vi "Accel Sensitivity.vi"(8 "error in (no error)":errorcluster, 11 "Accel Sensitivities":dbl[](array[numeric])) -> (0 "error out":errorcluster)   [LabVIEW 2018, in "PC UDP Writer.lvlib"]
doc: "This subVI enqueues the named action in to the communications queue along with the input data."
uses:
  PC UDP Writer.lvlib
  Private Controls/Module Data.ctl
  Private Controls/Module Action.ctl
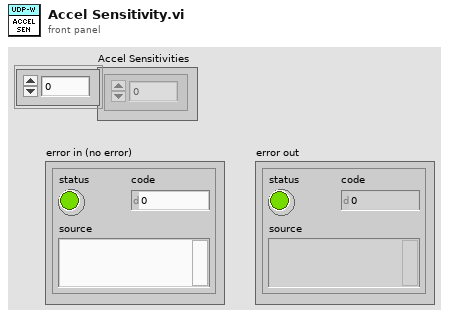
[diagram p1: front panel]
types:
  T1 = typedef "PC UDP Writer.lvlib/Module Data.ctl" = cluster{"Data":variant, "Action":T2}
  T2 = typedef "PC UDP Writer.lvlib/Module Action.ctl" = enum8{"Init", "Waterfall Select", "Bleed Fuel", "Fuel Pressure Reg", "ECS Demand", "Accel Sensitivities", "Accel Filters", "Shunt Relay", "APU Setup", "APU and ECU Control", "APU Start", "Write", "Error", "Exit"}
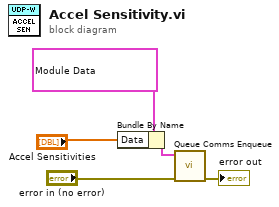
[diagram p0: block diagram]
diagram:
  n1 = Bundle By Name(cluster=T1 {"Data"=variant, "Action"=enum."Accel Sensitivities"} ("element"), "Data"="Accel Sensitivities") -> (w2:T1)
  n2 = call "Queue Comms Enqueue.vi"("error in (no error)"="error in (no error)", "element"=w2) -> ("error out"=→"error out":errorcluster)  [unwired: 9 in]
